vi "image_processing.vi"(5 "NG_rules":T3, 7 "parameter":T2={"image imshow"=FALSE, "side length (mm)"=0.0, "Main Range (Threshold)"={"Lower value"=73.0, "Upper value"=255.0}, "side velocity threshold"=0.0, "Sub Range (Threshold)"={"Lower value"=73.0, "Upper value"=255.0}, "close kernel size"=0.0, "open kernel size"=0.0, "side angle offest (threshold)"=0.0}, 11 "image":T1(plugin-control)) -> (0 "PASS":bool, 2 "NG code":dbl, 3 "display image":T1(plugin-control), 4 "angle offset":dbl)   [LabVIEW 2017]
uses:
  <vilib>/vision/NI_Vision_Development_Module.lvlib
panel:
  out "side angle offest":dbl
  out "side length (mm)":dbl
  out "ratio (cutting offest)":dbl
  out "damaged (mil)":dbl
  out "glitch (mil)":dbl
  out "open kernel size":dbl
  out "close kernel size":dbl
  in  "side velocity threshold":dbl
  out "Main Range (Threshold)":cluster{"Lower value":sgl, "Upper value":sgl}={"Lower value"=73.0, "Upper value"=255.0}
  out "image imshow":bool
  out "time image processing":u32
  out "time load image":u32
  out "Y Resolution":i32
  out "X Resolution":i32
  out "black image":T1(plugin-control)
  out "buffer image":T1(plugin-control)
  out "Sub Range (Threshold)":cluster{"Lower value":sgl, "Upper value":sgl}={"Lower value"=73.0, "Upper value"=255.0}
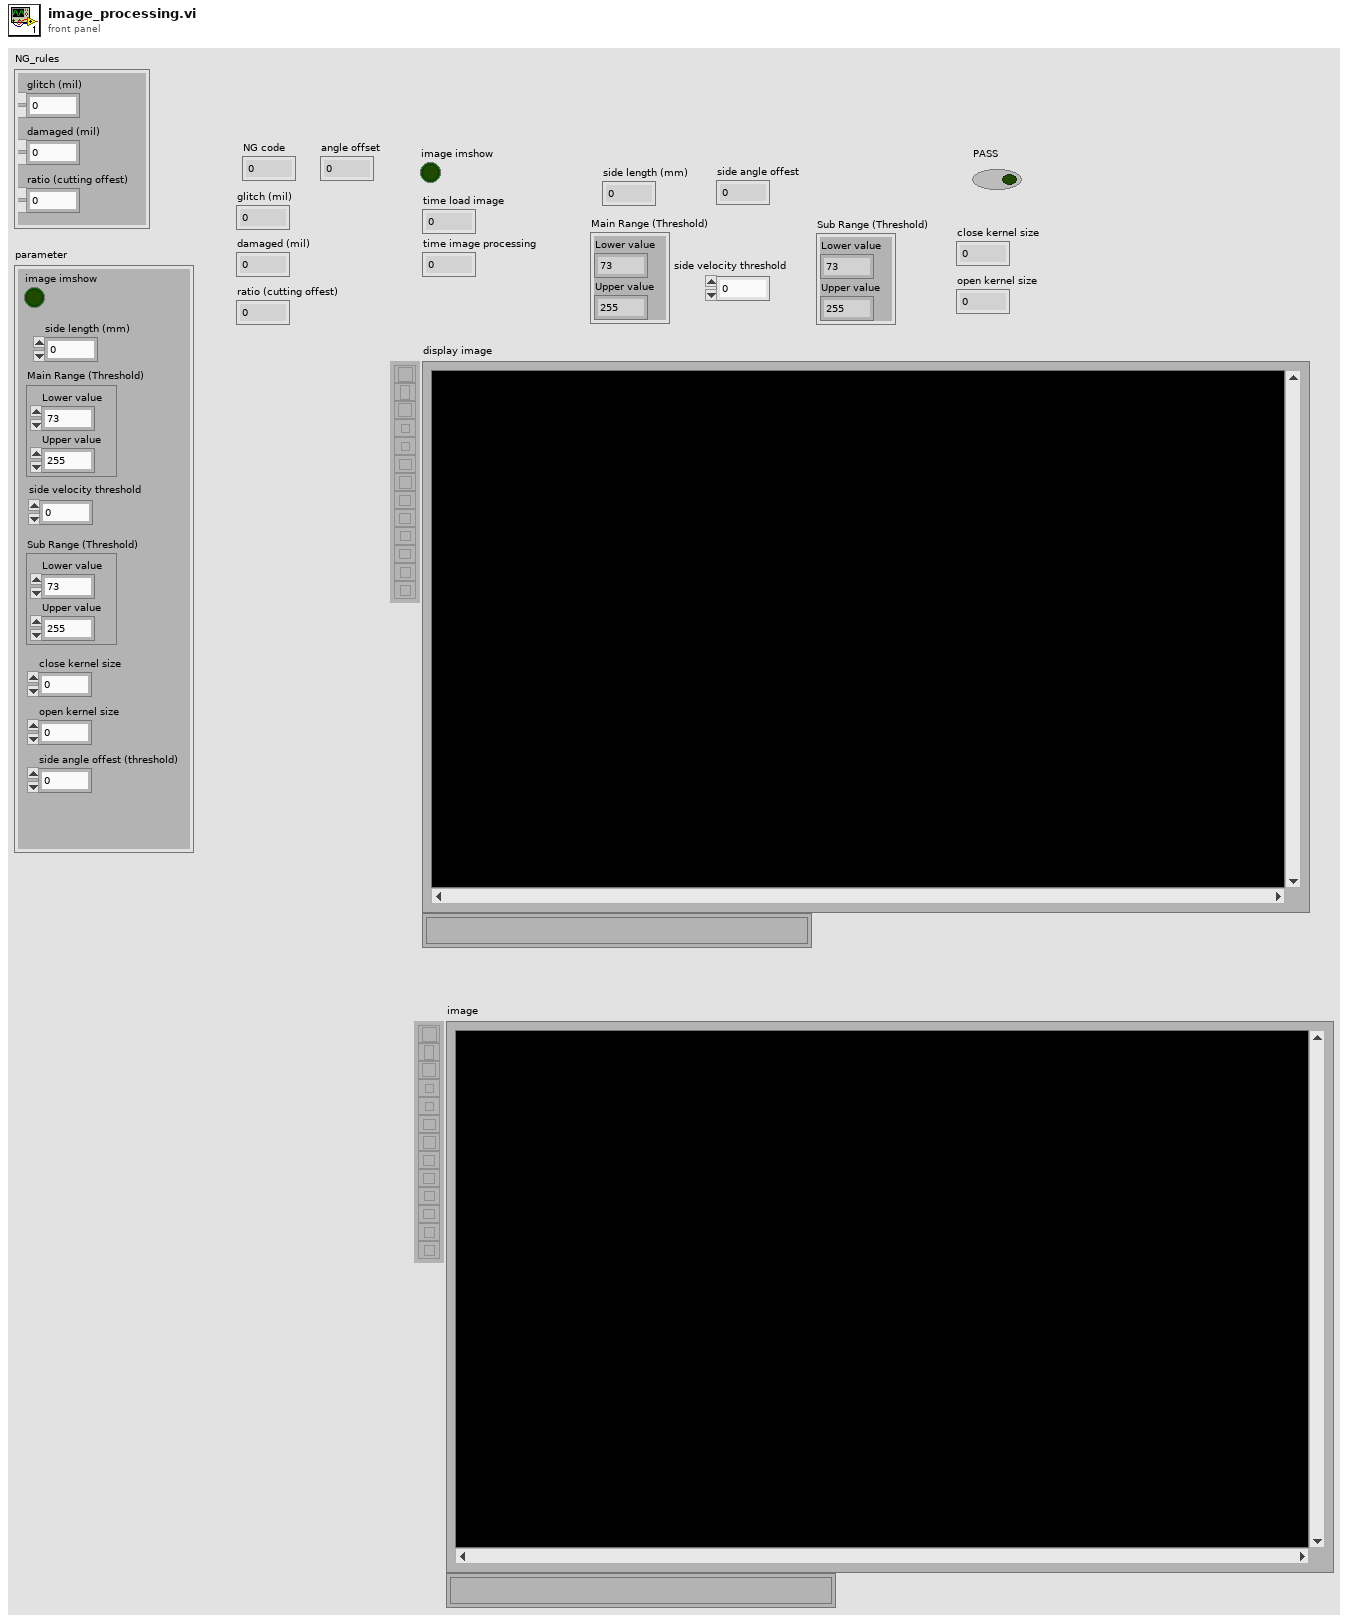
[diagram p1: front panel]
types:
  T1 = typedef "IMAQ Image.ctl" = refnum<image>
  T2 = cluster{"image imshow":bool, "side length (mm)":dbl, "Main Range (Threshold)":cluster{"Lower value":sgl, "Upper value":sgl}, "side velocity threshold":dbl, "Sub Range (Threshold)":cluster{"Lower value":sgl, "Upper value":sgl}, "close kernel size":dbl, "open kernel size":dbl, "side angle offest (threshold)":dbl}
  T3 = cluster{"glitch (mil)":dbl, "damaged (mil)":dbl, "ratio (cutting offest)":dbl}
  T4 = cluster{"Desired Font (Application)":enum16{"User-specified Font", "Application Font", "System Font", "Dialog Font"}, "[User-specified Font]":cluster{"Font Name":string, "Size":i16, "Strikeout?":bool, "Italic?":bool, "Underline?":bool, "Outline?":bool, "Shadow?":bool, "Bold?":bool, "Rotation Angle":dbl}, "Horizontal Alignment":i16, "Vertical Alignment":i16}
  T5 = enum32{"AutoM", "Close", "Dilate", "Erode", "Gradient", "Gradient out", "Gradient in", "Hit miss", "Open", "PClose", "POpen", "Thick", "Thin"}
  T6 = cluster{"Sigma":sgl, "HThresh":sgl, "LThres":sgl, "WindowSize":i32}
  T7 = cluster{"Number of Points":i32, "Open/Closed":i32, "Weight":dbl, "Contour Points":cluster{"X":dbl, "Y":dbl, "Curvature":dbl, "X Displacement":dbl, "Y Displacement":dbl}[]}[]
  T8 = cluster{"Left":i32, "Top":i32, "Right":i32, "Bottom":i32}
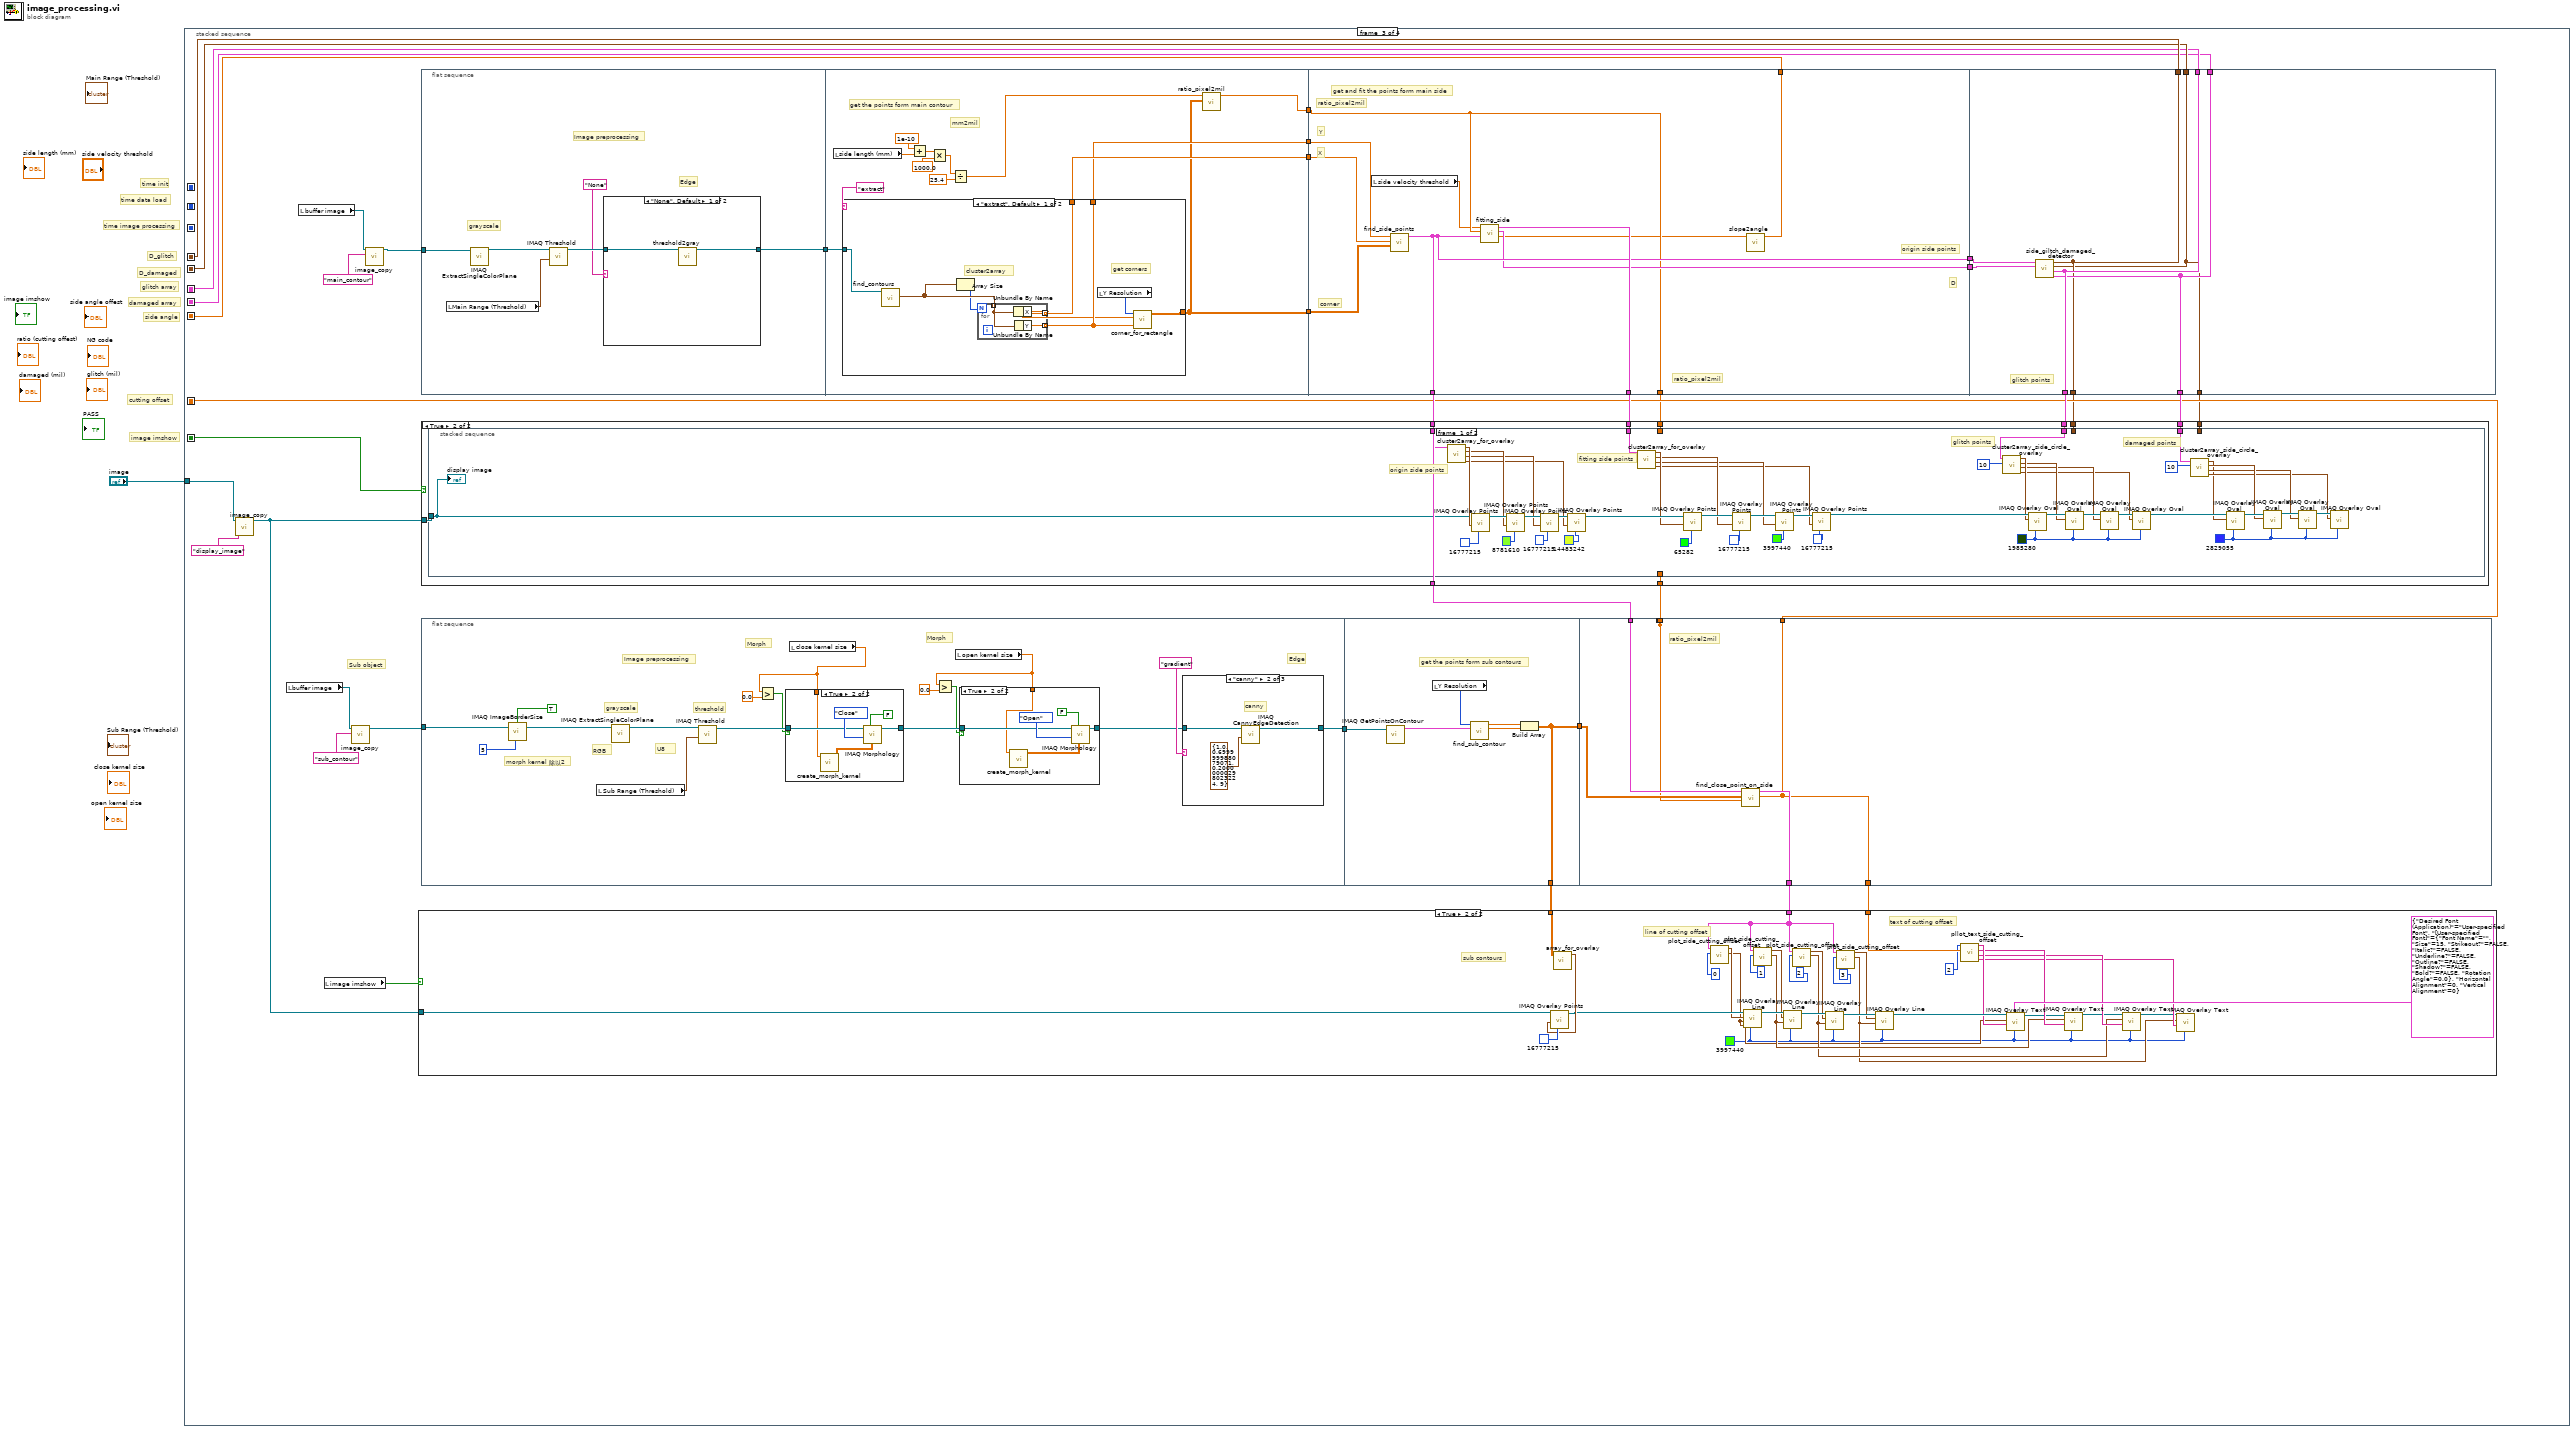
[diagram p0: block diagram]
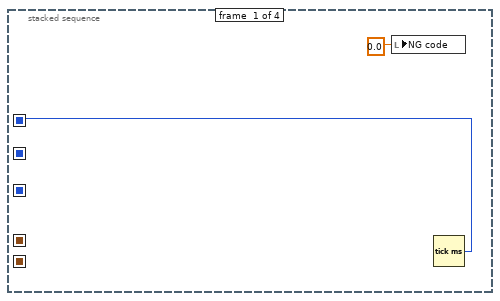
[diagram p2: hidden frame]
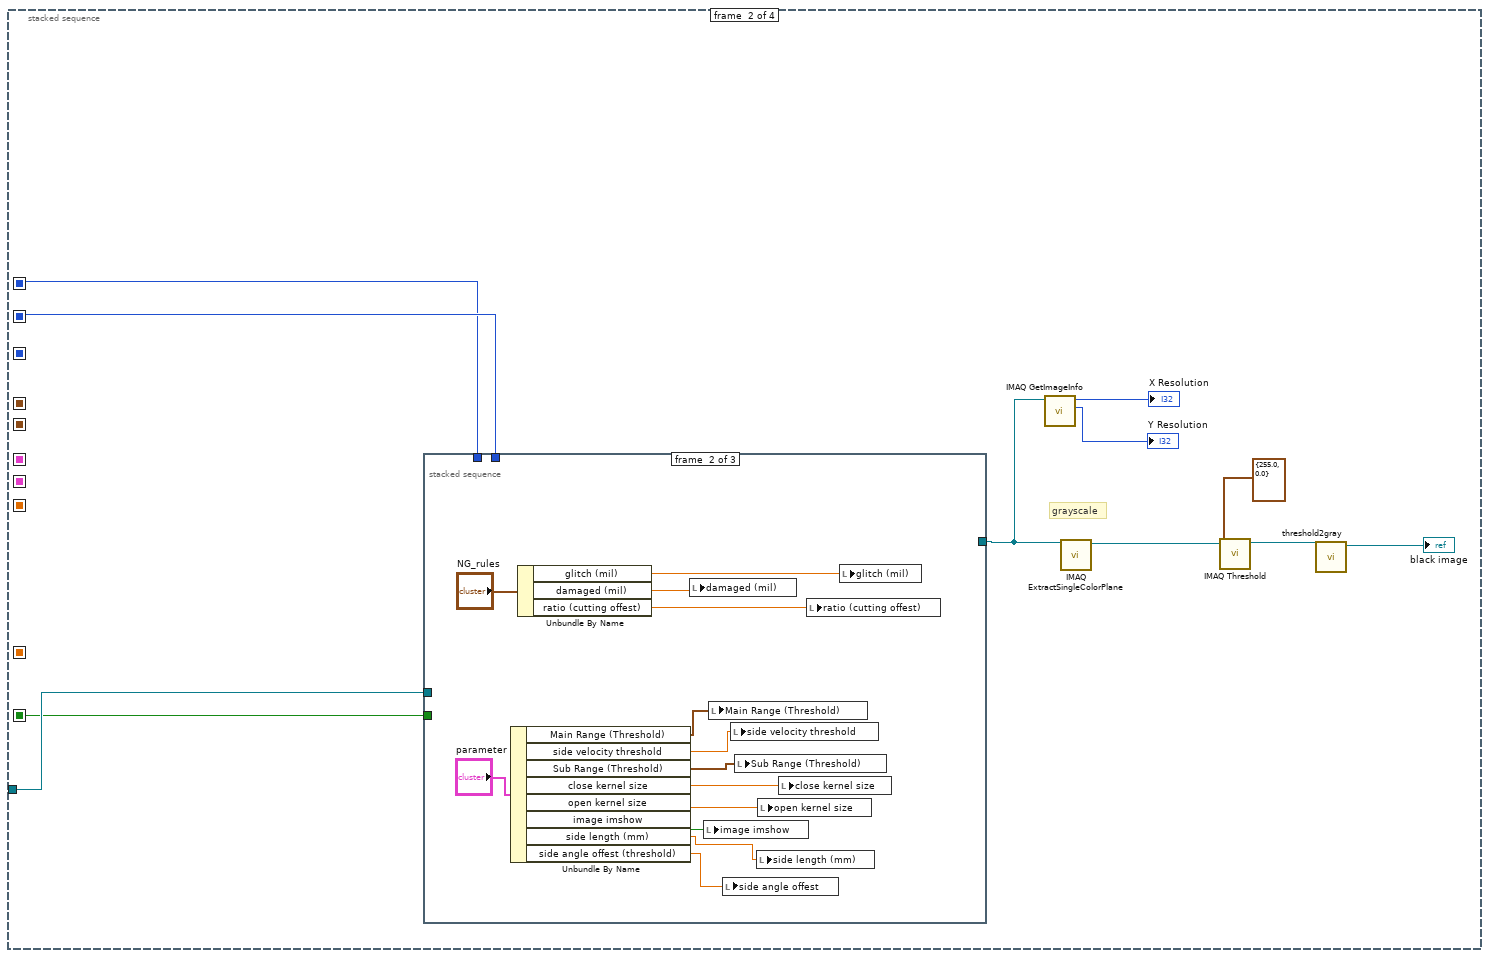
[diagram p3: hidden frame]
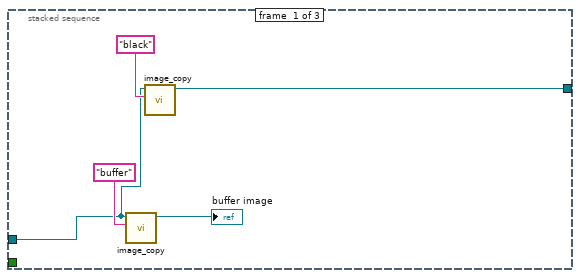
[diagram p4: hidden frame]
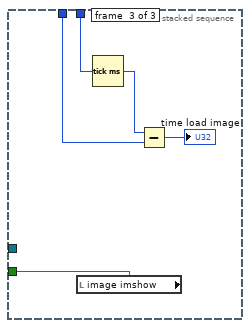
[diagram p5: hidden frame]
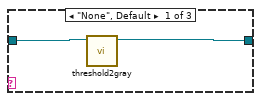
[diagram p9: hidden frame]
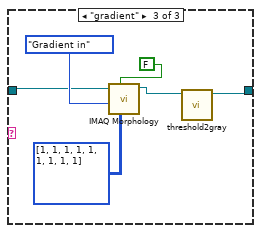
[diagram p10: hidden frame]
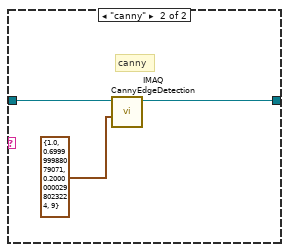
[diagram p11: hidden frame]
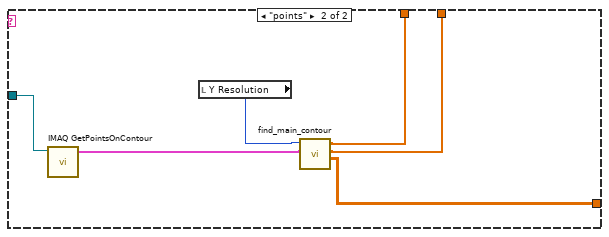
[diagram p12: hidden frame]
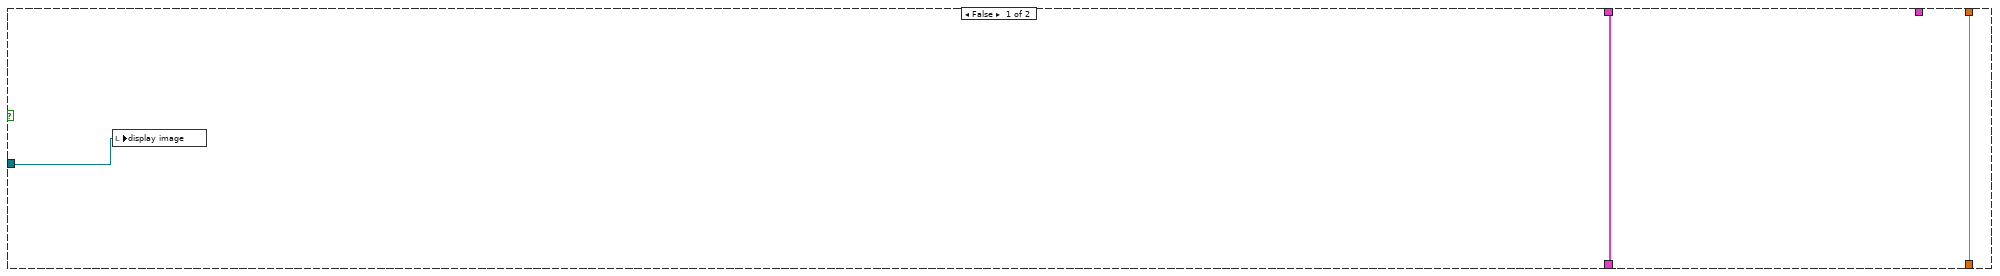
[diagram p13: hidden frame]
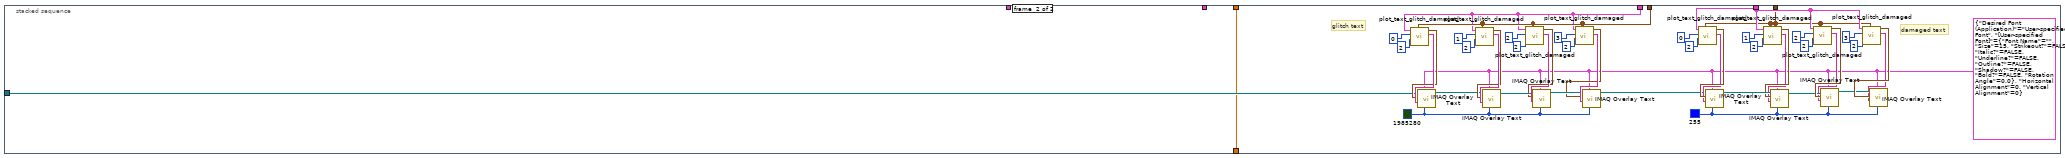
[diagram p14: hidden frame]
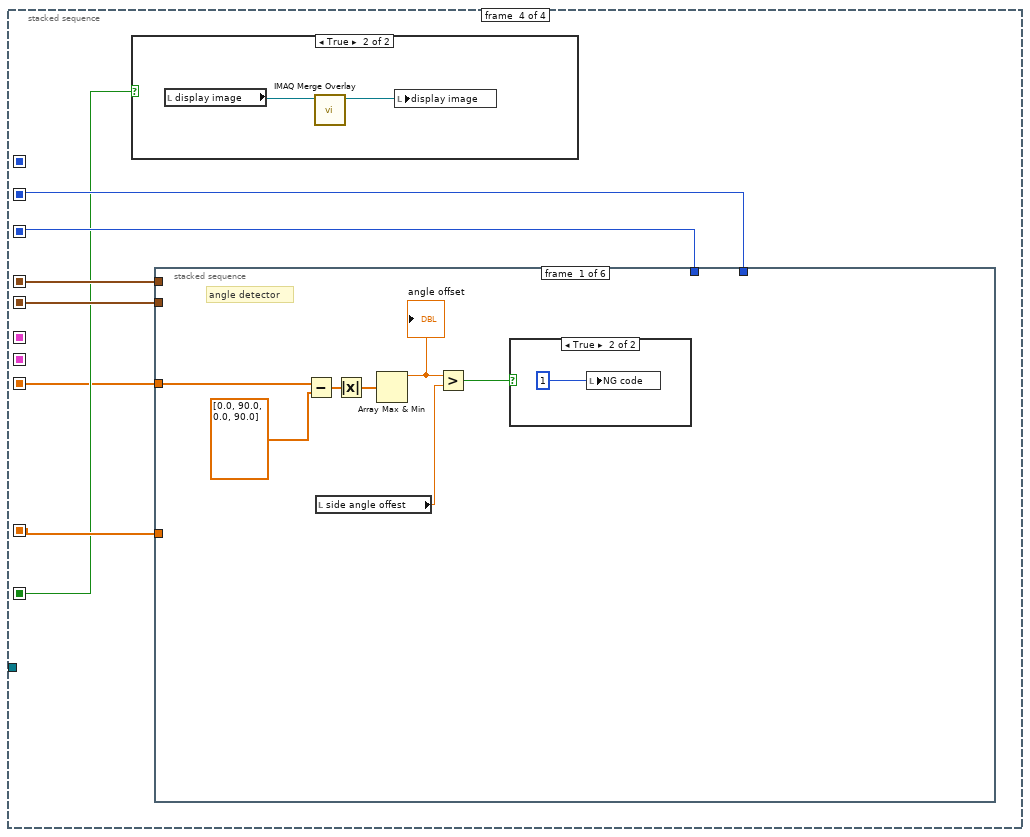
[diagram p15: hidden frame]
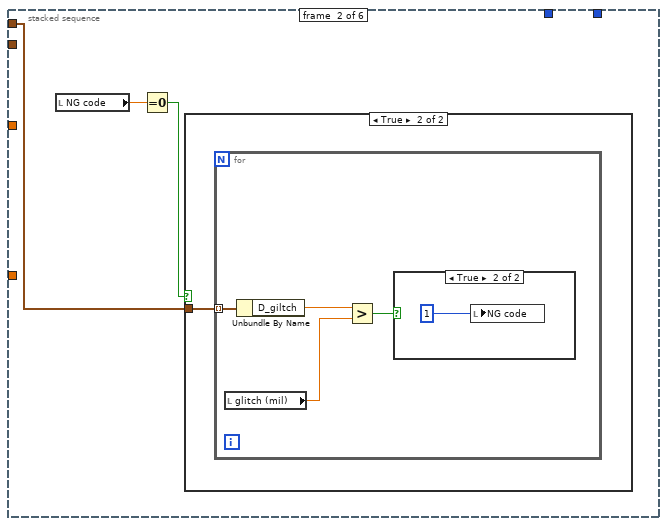
[diagram p18: hidden frame]
diagram:
  # "side angle"
  # "image imshow"
  # "cutting offset"
  # "damaged array"
  # "glitch array"
  # "D_damaged"
  # "D_glitch"
  # "time image processing"
  # "time data load"
  # "time init"
  n1 = stacked-sequence {
    seq-local: [w3 _ _ _] -> [_ w7 _ _]
    seq-local: [_ w8 _ _] -> [_ _ _ w330]
    seq-local: [_ _ _ w331] -> [_ _ _ _]
    seq-local: [_ _ w49 _] -> [_ _ _ w329]
    seq-local: [_ _ w48 _] -> [_ _ _ w328]
    seq-local: [_ _ w47 _] -> [_ _ _ _]
    seq-local: [_ _ w46 _] -> [_ _ _ _]
    seq-local: [_ _ w44 _] -> [_ _ _ w327]
    seq-local: [_ w4 _ _] -> [_ _ w38 w326]
    seq-local: [_ _ w37 _] -> [_ _ _ w325]
    tunnel: "image" -> [_ w9 w56 _]
    frame #0 {
      n2 = local write "NG code"(0.0 ("NG code")) -> ()
      n3 = Tick Count (ms)() -> (millisecond timer value=w3:u32)
    }
    frame #1 {
      # "grayscale"
      n4 = stacked-sequence {
        tunnel: [w17 _ _] -> w12
        tunnel: w9 -> [w16 _ _]
        tunnel: [_ _ w36] -> w8
        tunnel: w7 -> [_ _ w35]
        tunnel: [_ _ w33] -> w4
        frame #0 {
          n5 = call "image_copy.vi"("buffer name"="buffer" ("Image Name"), "image in"=w16) -> ("imgae out"=→"buffer image":T1)  [unwired: 9 in]
          n6 = call "image_copy.vi"("buffer name"="black" ("Image Name"), "image in"=w16) -> ("imgae out"=w17:T1)  [unwired: 9 in]
        }
        frame #1 {
          n7 = Unbundle By Name("parameter") -> ("Main Range (Threshold)"=w27:cluster{"Lower value":sgl, "Upper value":sgl}, "side velocity threshold"=w26:dbl, "Sub Range (Threshold)"=w25:cluster{"Lower value":sgl, "Upper value":sgl}, "close kernel size"=w24:dbl, "open kernel size"=w23:dbl, "image imshow"=w22:bool, "side length (mm)"=w21:dbl, "side angle offest (threshold)"=w20:dbl)
          n8 = Unbundle By Name("NG_rules") -> ("glitch (mil)"=w31:dbl, "damaged (mil)"=w30:dbl, "ratio (cutting offest)"=w29:dbl)
          n9 = local write "damaged (mil)"(w30) -> ()
          n10 = local write "image imshow"(w22) -> ()
          n11 = local write "Main Range (Threshold)"(w27) -> ()
          n12 = local write "side angle offest"(w20) -> ()
          n13 = local write "side velocity threshold"(w26) -> ()
          n14 = local write "Sub Range (Threshold)"(w25) -> ()
          n15 = local write "side length (mm)"(w21) -> ()
          n16 = local write "open kernel size"(w23) -> ()
          n17 = local write "close kernel size"(w24) -> ()
          n18 = local write "ratio (cutting offest)"(w29) -> ()
          n19 = local write "glitch (mil)"(w31) -> ()
        }
        frame #2 {
          n20 = local read "image imshow"() -> (w33:bool)
          n21 = Tick Count (ms)() -> (millisecond timer value=w36:u32)
          n22 = Subtract(x=w36, y=w35) -> (x-y=→"time load image":u32)
        }
      }
      n23 = call "IMAQ GetImageInfo"("Image"=w12) -> ("Y Resolution"=→"Y Resolution":i32, "X Resolution"=→"X Resolution":i32)  [unwired: 3 in, 6 out]
      n24 = call "IMAQ ExtractSingleColorPlane"("Image Src"=w12) -> ("Image Dst Out"=w14:T1)  [unwired: 3 in, 7 out]
      n25 = call "IMAQ Threshold"("Range"=cluster{"Lower value":sgl, "Upper value":sgl} {"Lower value"=255.0, "Upper value"=0.0}, "Image Src"=w14) -> ("Image Dst Out"=w6:T1)  [unwired: 4 in, 5 out]
      n26 = call "threshold2gray.vi"("threshold image"=w6) -> ("grayscale image"=→"black image":T1)  [unwired: 10 in]
    }
    frame #2 {
      # "Sub object"
      n27 = call "image_copy.vi"("buffer name"="display_image" ("Image Name"), "image in"=w56) -> ("imgae out"=w55:T1)  [unwired: 9 in]
      n28 = local read "buffer image"() -> (w65:T1)
      n29 = local read "buffer image"() -> (w73:T1)
      n30 = local read "image imshow"() -> (w52:bool)
      n31 = call "image_copy.vi"("buffer name"="sub_contour" ("Image Name"), "image in"=w65) -> ("imgae out"=w64:T1)  [unwired: 9 in]
      n32 = call "image_copy.vi"("buffer name"="main_contour" ("Image Name"), "image in"=w73) -> ("imgae out"=w72:T1)  [unwired: 9 in]
      n33 = case shown="True" w52 {
        tunnel: w55 -> [_ w75]
        tunnel: w54 -> [_ w105]
        tunnel: w53 -> [_ w97]
        tunnel: w43 -> [_ w90]
        frame False {
        }
        frame True {
          w76 = u32 3997440 ("Text Color (black)")
          # "text of cutting offset"
          # "line of cutting offset"
          # "sub contours"
          n34 = call "array_for_overlay.vi"("Array in"=w105) -> ("Array out"=w106:cluster{"X":i32, "Y":i32}[])  [unwired: 10 in]
          n35 = call "IMAQ Overlay Points"("Color"=u32 16777215, "Array of Points"=w106, "Image"=w75) -> ("Image Out"=w104:T1)  [unwired: 7 in, 1 out]
          n36 = call "plot_side_cutting_offset.vi"("index"=0, "coord cluster"=w97) -> ("End Point out"=w77:cluster{"X":i32, "Y":i32}, "Start Point out"=w87:cluster{"X":i32, "Y":i32})  [unwired: 8 in]
          n37 = call "IMAQ Overlay Line"("Color"=w76, "End Point"=w77, "Start Point"=w87, "Image"=w104) -> ("Image Out"=w103:T1)  [unwired: 6 in, 1 out]
          n38 = call "plot_side_cutting_offset.vi"("index"=1, "coord cluster"=w97) -> ("End Point out"=w80:cluster{"X":i32, "Y":i32}, "Start Point out"=w92:cluster{"X":i32, "Y":i32})  [unwired: 8 in]
          n39 = call "IMAQ Overlay Line"("Color"=w76, "End Point"=w80, "Start Point"=w92, "Image"=w103) -> ("Image Out"=w102:T1)  [unwired: 6 in, 1 out]
          n40 = call "plot_side_cutting_offset.vi"("index"=2, "coord cluster"=w97) -> ("End Point out"=w79:cluster{"X":i32, "Y":i32}, "Start Point out"=w93:cluster{"X":i32, "Y":i32})  [unwired: 8 in]
          n41 = call "IMAQ Overlay Line"("Color"=w76, "End Point"=w79, "Start Point"=w93, "Image"=w102) -> ("Image Out"=w101:T1)  [unwired: 6 in, 1 out]
          n42 = call "plot_side_cutting_offset.vi"("index"=3, "coord cluster"=w97) -> ("End Point out"=w78:cluster{"X":i32, "Y":i32}, "Start Point out"=w94:cluster{"X":i32, "Y":i32})  [unwired: 8 in]
          n43 = call "IMAQ Overlay Line"("Color"=w76, "End Point"=w78, "Start Point"=w94, "Image"=w101) -> ("Image Out"=w95:T1)  [unwired: 6 in, 1 out]
          n44 = call "pllot_text_side_cutting_offset.vi"("D cutting offset array"=w90, "precision"=2 ("index")) -> ("Left side length"=w84:string, "Bottom side length"=w85:string, "Right side length"=w86:string, "Top side length"=w88:string)  [unwired: 6 in]
          n45 = call "IMAQ Overlay Text"("Text Color (black)"=w76, "Font, Size & Style"=T4 {"Desired Font (Application)"=enum."User-specified Font", "[User-specified Font]"={"Font Name"="", "Size"=15, "Strikeout?"=FALSE, "Italic?"=FALSE, "Underline?"=FALSE, "Outline?"=FALSE, "Shadow?"=FALSE, "Bold?"=FALSE, "Rotation Angle"=0.0}, "Horizontal Alignment"=0, "Vertical Alignment"=0}, "String"=w88, "Origin"=w77, "Image"=w95) -> ("Image Out"=w83:T1)  [unwired: 5 in, 1 out]
          n46 = call "IMAQ Overlay Text"("Text Color (black)"=w76, "String"=w86, "Origin"=w80, "Image"=w83) -> ("Image Out"=w82:T1)  [unwired: 6 in, 1 out]
          n47 = call "IMAQ Overlay Text"("Text Color (black)"=w76, "String"=w85, "Origin"=w79, "Image"=w82) -> ("Image Out"=w81:T1)  [unwired: 6 in, 1 out]
          n48 = call "IMAQ Overlay Text"("Text Color (black)"=w76, "String"=w84, "Origin"=w78, "Image"=w81) -> ()  [unwired: 6 in, 2 out]
        }
      }
      n49 = flat-sequence {
        tunnel: w72 -> [w166]
        tunnel: [w163] -> w71
        tunnel: w71 -> [w183]
        tunnel: [w177] -> w70
        tunnel: [w182] -> w68
        tunnel: [w181] -> w67
        tunnel: [w175] -> w59
        tunnel: w70 -> [w210]
        tunnel: [w206] -> w69
        tunnel: w68 -> [w209]
        tunnel: w67 -> [w208]
        tunnel: [w207] -> w62
        tunnel: w59 -> [w204]
        tunnel: [w206] -> w51
        tunnel: [w205] -> w50
        tunnel: [w204] -> w40
        tunnel: [w201] -> w37
        tunnel: [w214] -> w61
        tunnel: [w213] -> w60
        tunnel: w51 -> [w216]
        tunnel: w50 -> [w215]
        tunnel: [w214] -> w47
        tunnel: [w213] -> w46
        tunnel: [w212] -> w49
        tunnel: [w211] -> w48
        tunnel: [w212] -> w42
        tunnel: [w211] -> w41
        frame #0 {
          # "Image preprocessing"
          # "grayscale"
          # "Edge"
          n50 = local read "Main Range (Threshold)"() -> (w161:cluster{"Lower value":sgl, "Upper value":sgl})
          n51 = call "IMAQ ExtractSingleColorPlane"("Image Src"=w166) -> ("Image Dst Out"=w165:T1)  [unwired: 3 in, 7 out]
          n52 = call "IMAQ Threshold"("Range"=w161, "Image Src"=w165) -> ("Image Dst Out"=w164:T1)  [unwired: 4 in, 5 out]
          n53 = case shown="\"None\", Default" "None" {
            tunnel: [w167 w171] -> w163
            tunnel: w164 -> [w168 w170]
            frame "None", Default {
              n54 = call "threshold2gray.vi"("threshold image"=w168) -> ("grayscale image"=w167:T1)  [unwired: 10 in]
            }
            frame "canny" {
              # "canny"
              n55 = call "IMAQ CannyEdgeDetection"("Image Src"=w170, "Filter Parameters"=T6 {"Sigma"=1.0, "HThresh"=0.7, "LThres"=0.2, "WindowSize"=9}) -> ("Image Dst Out"=w171:T1)  [unwired: 2 in, 5 out]
            }
          }
        }
        frame #1 {
          # "mm2mil"
          # "get the points form main contour"
          n56 = local read "side length (mm)"() -> (w172:dbl)
          n57 = case shown="\"extract\", Default" "extract" {
            tunnel: w183 -> [w187 w200]
            tunnel: [w188 w195] -> w177
            tunnel: [w186 w196] -> w181
            tunnel: [w185 w197] -> w182
            frame "extract", Default {
              # "get corners"
              # "cluster2array"
              n58 = call "find_contours.vi"("image in"=w187) -> ("Source Image Points"=w191:cluster{"X":dbl, "Y":dbl}[])  [unwired: 9 in, 1 out]
              n59 = Array Size(array=w191) -> (size(s)=w189:i32)
              n60 = for {
                N: w189 -> [_]
                tunnel: w191 -> [w193] mode=indexing
                tunnel: [w194] -> w185 mode=indexing
                tunnel: [w192] -> w186 mode=indexing
                n61 = Unbundle By Name(w193) -> ("X"=w194:dbl)
                n62 = Unbundle By Name(w193) -> ("Y"=w192:dbl)
              }
              n63 = local read "Y Resolution"() -> (w190:i32)
              n64 = call "corner_for_rectangle.vi"("Y"=w186, "X"=w185, "Y Resolution"=w190) -> ("corner"=w188:dbl[][])  [unwired: 7 in, 1 out]
            }
            frame "points" {
              n65 = call "IMAQ GetPointsOnContour"("Image (Edge Image)"=w200) -> ("Segment Information"=w198:T7)  [unwired: 3 in, 2 out]
              n66 = local read "Y Resolution"() -> (w199:i32)
              n67 = call "find_main_contour.vi"("Segment Information"=w198, "Y Resolution"=w199) -> ("max corner"=w195:dbl[][], "Y"=w196:dbl[], "X"=w197:dbl[])  [unwired: 7 in]
            }
          }
          n68 = Add(x=1e-10, y=w172) -> (x+y=w173:dbl)
          n69 = Multiply(x=w173, y=1000.0) -> (x*y=w179:dbl)
          n70 = Divide(x=w179, y=25.4) -> (x/y=w176:dbl)
          n71 = call "ratio_pixel2mil.vi"("max corner in"=w177, "side length (mm)"=w176) -> ("ratio"=w175:dbl)  [unwired: 9 in]
        }
        frame #2 {
          # "ratio_pixel2mil"
          # "origin side points"
          # "D"
          # "corner"
          # "X"
          # "Y"
          # "ratio_pixel2mil"
          # "get and fit the points form main side"
          n72 = local read "side velocity threshold"() -> (w203:dbl)
          n73 = call "find_side_points.vi"("corner"=w210, "X  coords array"=w209, "Y coords array"=w208) -> ("side of clusters"=w206:cluster{"Array out":dbl[][]}[])  [unwired: 8 in]
          n74 = call "fitting_side.vi"("side of clusters"=w206, "ratio"=w204, "side velocity threshold"=w203) -> ("slope array"=w202:dbl[], "D of clusters"=w205:cluster{"D":ext[]}[], "fitting clusters"=w207:cluster{"fitting array":dbl[][]}[])  [unwired: 6 in]
          n75 = call "slope2angle.vi"("slope array"=w202) -> ("x/y"=w201:dbl[])  [unwired: 10 in]
        }
        frame #3 {
          # "glitch points"
          n76 = call "side_giltch_damaged_detector.vi"("D of clusters"=w215, "side of clusters"=w216) -> ("damaged clusters"=w213:cluster{"damaged coord":dbl[]}[], "giltch of clusters"=w214:cluster{"giltch_coord":dbl[]}[], "D damaged of clusters"=w211:cluster{"D_damaged":ext}[], "D giltch of clusters"=w212:cluster{"D_giltch":ext}[])  [unwired: 6 in]
        }
      }
      n77 = flat-sequence {
        tunnel: w64 -> [w121]
        tunnel: [w117] -> w63
        tunnel: w63 -> [w155]
        tunnel: [w150] -> w58
        tunnel: [w150] -> w54
        tunnel: w58 -> [w160]
        tunnel: [w159] -> w53
        tunnel: w45 -> [w158]
        tunnel: [w156] -> w44
        tunnel: [w156] -> w43
        tunnel: [w157] -> _
        tunnel: w39 -> [w157]
        frame #0 {
          # "Morph"
          # "Image preprocessing"
          # "Morph"
          # "morph kernel 除以2"
          # "Edge"
          # "U8"
          # "RGB"
          # "threshold"
          # "grayscale"
          n78 = call "IMAQ ImageBorderSize"("Get/Set Status? (Set)"=TRUE, "Image"=w121, "Image border size in"=5) -> ("Image Out"=w120:T1)  [unwired: 1 in, 2 out]
          n79 = local read "Sub Range (Threshold)"() -> (w110:cluster{"Lower value":sgl, "Upper value":sgl})
          n80 = call "IMAQ ExtractSingleColorPlane"("Image Src"=w120) -> ("Image Dst Out"=w124:T1)  [unwired: 3 in, 7 out]
          n81 = call "IMAQ Threshold"("Range"=w110, "Image Src"=w124) -> ("Image Dst Out"=w122:T1)  [unwired: 4 in, 5 out]
          n82 = local read "close kernel size"() -> (w109:dbl)
          n83 = Greater?(x=w109, y=0.0) -> (0:w114:bool)
          n84 = case shown="True" w114 {
            tunnel: w122 -> [w132 w137]
            tunnel: [w132 w136] -> w115
            tunnel: w109 -> [_ w135]
            frame False {
            }
            frame True {
              n85 = call "create_morph_kernel.vi"("kernel size"=w135) -> ("kernel"=w134:dbl[][])  [unwired: 10 in]
              n86 = call "IMAQ Morphology"("Structuring Element"=w134, "Square/Hexa (Square)"=FALSE, "Operation"=T5."Close", "Image Src"=w137) -> ("Image Dst Out"=w136:T1)  [unwired: 3 in, 4 out]
            }
          }
          n87 = local read "open kernel size"() -> (w108:dbl)
          n88 = Greater?(x=w108, y=0.0) -> (0:w111:bool)
          n89 = case shown="True" w111 {
            tunnel: [w125 w130] -> w116
            tunnel: w115 -> [w125 w129]
            tunnel: w108 -> [_ w126]
            frame False {
            }
            frame True {
              n90 = call "create_morph_kernel.vi"("kernel size"=w126) -> ("kernel"=w127:dbl[][])  [unwired: 10 in]
              n91 = call "IMAQ Morphology"("Structuring Element"=w127, "Square/Hexa (Square)"=FALSE, "Operation"=T5."Open", "Image Src"=w129) -> ("Image Dst Out"=w130:T1)  [unwired: 3 in, 4 out]
            }
          }
          n92 = case shown="\"canny\"" "gradient" {
            tunnel: [w139 w143 w144] -> w117
            tunnel: w116 -> [w140 w142 w146]
            frame "None", Default {
              n93 = call "threshold2gray.vi"("threshold image"=w140) -> ("grayscale image"=w139:T1)  [unwired: 10 in]
            }
            frame "canny" {
              # "canny"
              n94 = call "IMAQ CannyEdgeDetection"("Image Src"=w142, "Filter Parameters"=T6 {"Sigma"=1.0, "HThresh"=0.7, "LThres"=0.2, "WindowSize"=9}) -> ("Image Dst Out"=w143:T1)  [unwired: 2 in, 5 out]
            }
            frame "gradient" {
              n95 = call "IMAQ Morphology"("Structuring Element"=i32[][] [[1, 1, 1], [1, 1, 1], [1, 1, 1]], "Square/Hexa (Square)"=FALSE, "Operation"=T5."Gradient in", "Image Src"=w146) -> ("Image Dst Out"=w145:T1)  [unwired: 3 in, 4 out]
              n96 = call "threshold2gray.vi"("threshold image"=w145) -> ("grayscale image"=w144:T1)  [unwired: 10 in]
            }
          }
        }
        frame #1 {
          # "get the points form sub contours"
          n97 = call "IMAQ GetPointsOnContour"("Image (Edge Image)"=w155) -> ("Segment Information"=w154:T7)  [unwired: 3 in, 2 out]
          n98 = local read "Y Resolution"() -> (w153:i32)
          n99 = call "find_sub_contour.vi"("Segment Information"=w154, "Y Resolution"=w153) -> ("Y"=w151:dbl[], "X"=w152:dbl[])  [unwired: 8 in]
          n100 = Build Array(w152, w151) -> (w150:dbl[][])
        }
        frame #2 {
          # "ratio_pixel2mil"
          n101 = call "find_close_point_on_side.vi"("ratio_pixel2mil"=w157, "Array"=w160, "fitting clusters"=w158) -> ("D cutting offset array"=w156:ext[], "coord cluster"=w159:cluster{dbl[][]}[])  [unwired: 7 in]
        }
      }
      n102 = case shown="True" w38 {
        tunnel: w55 -> [w218 w228]
        tunnel: w69 -> [w217 w220]
        tunnel: w62 -> [_ w225]
        tunnel: w61 -> [_ w226]
        tunnel: w60 -> [_ w227]
        tunnel: [w217 w220] -> w45
        tunnel: w42 -> [_ w224]
        tunnel: w41 -> [_ w223]
        tunnel: w40 -> [w219 w222]
        tunnel: [w219 w221] -> w39
        frame False {
          n103 = local write "display image"(w218) -> ()
        }
        frame True {
          n104 = stacked-sequence {
            tunnel: w228 -> [w229 w320]
            tunnel: w220 -> [w251 _]
            tunnel: w227 -> [w236 w283]
            tunnel: w226 -> [w231 w305]
            tunnel: w225 -> [w230 _]
            tunnel: w224 -> [_ w307]
            tunnel: w223 -> [_ w282]
            tunnel: w222 -> [_ w278]
            tunnel: [_ w278] -> w221
            frame #0 {
              w253 = u32 2829055 ("Color")
              w254 = u32 1985280 ("Color")
              # "damaged points"
              # "glitch points"
              # "fitting side points"
              # "origin side points"
              n105 = call "cluster2array_for_overlay.vi"("side of clusters"=w251) -> ("Left side points"=w247:cluster{"X":i32, "Y":i32}[], "Bottom side points"=w248:cluster{"X":i32, "Y":i32}[], "Right side points"=w249:cluster{"X":i32, "Y":i32}[], "Top side points"=w250:cluster{"X":i32, "Y":i32}[])  [unwired: 7 in]
              n106 = call "IMAQ Overlay Points"("Color"=u32 16777215, "Array of Points"=w250, "Image"=w229) -> ("Image Out"=w273:T1)  [unwired: 7 in, 1 out]
              n107 = call "IMAQ Overlay Points"("Color"=u32 8781610, "Array of Points"=w249, "Image"=w273) -> ("Image Out"=w275:T1)  [unwired: 7 in, 1 out]
              n108 = call "IMAQ Overlay Points"("Color"=u32 16777215, "Array of Points"=w248, "Image"=w275) -> ("Image Out"=w274:T1)  [unwired: 7 in, 1 out]
              n109 = call "IMAQ Overlay Points"("Color"=u32 14483242, "Array of Points"=w247, "Image"=w274) -> ("Image Out"=w262:T1)  [unwired: 7 in, 1 out]
              n110 = call "cluster2array_for_overlay.vi"("side of clusters"=w230) -> ("Left side points"=w243:cluster{"X":i32, "Y":i32}[], "Bottom side points"=w244:cluster{"X":i32, "Y":i32}[], "Right side points"=w245:cluster{"X":i32, "Y":i32}[], "Top side points"=w246:cluster{"X":i32, "Y":i32}[])  [unwired: 7 in]
              n111 = call "IMAQ Overlay Points"("Color"=u32 65282, "Array of Points"=w246, "Image"=w262) -> ("Image Out"=w266:T1)  [unwired: 7 in, 1 out]
              n112 = call "IMAQ Overlay Points"("Color"=u32 16777215, "Array of Points"=w245, "Image"=w266) -> ("Image Out"=w264:T1)  [unwired: 7 in, 1 out]
              n113 = call "IMAQ Overlay Points"("Color"=u32 3997440, "Array of Points"=w244, "Image"=w264) -> ("Image Out"=w265:T1)  [unwired: 7 in, 1 out]
              n114 = call "IMAQ Overlay Points"("Color"=u32 16777215, "Array of Points"=w243, "Image"=w265) -> ("Image Out"=w252:T1)  [unwired: 7 in, 1 out]
              n115 = call "cluster2array_side_circle_overlay.vi"("radius"=10 ("index"), "giltch of clusters"=w231) -> ("Left side points"=w239:T8, "Bottom side points"=w240:T8, "Right side points"=w241:T8, "Top side points"=w242:T8)  [unwired: 6 in]
              n116 = call "IMAQ Overlay Oval"("Color"=w254, "Bounding Rectangle"=w242, "Image"=w252) -> ("Image Out"=w261:T1)  [unwired: 7 in, 1 out]
              n117 = call "IMAQ Overlay Oval"("Color"=w254, "Bounding Rectangle"=w241, "Image"=w261) -> ("Image Out"=w260:T1)  [unwired: 7 in, 1 out]
              n118 = call "IMAQ Overlay Oval"("Color"=w254, "Bounding Rectangle"=w240, "Image"=w260) -> ("Image Out"=w259:T1)  [unwired: 7 in, 1 out]
              n119 = call "IMAQ Overlay Oval"("Color"=w254, "Bounding Rectangle"=w239, "Image"=w259) -> ("Image Out"=w255:T1)  [unwired: 7 in, 1 out]
              n120 = call "cluster2array_side_circle_overlay.vi"("radius"=10 ("index"), "giltch of clusters"=w236) -> ("Left side points"=w233:T8, "Bottom side points"=w234:T8, "Right side points"=w235:T8, "Top side points"=w232:T8)  [unwired: 6 in]
              n121 = call "IMAQ Overlay Oval"("Color"=w253, "Bounding Rectangle"=w232, "Image"=w255) -> ("Image Out"=w256:T1)  [unwired: 7 in, 1 out]
              n122 = call "IMAQ Overlay Oval"("Color"=w253, "Bounding Rectangle"=w235, "Image"=w256) -> ("Image Out"=w257:T1)  [unwired: 7 in, 1 out]
              n123 = call "IMAQ Overlay Oval"("Color"=w253, "Bounding Rectangle"=w234, "Image"=w257) -> ("Image Out"=w258:T1)  [unwired: 7 in, 1 out]
              n124 = call "IMAQ Overlay Oval"("Color"=w253, "Bounding Rectangle"=w233, "Image"=w258) -> ()  [unwired: 7 in, 2 out]
              "display image" <- w229
            }
            frame #1 {
              w277 = u32 1985280 ("Color")
              w280 = u32 255 ("Text Color (black)")
              w281 = T4 {"Desired Font (Application)"=enum."User-specified Font", "[User-specified Font]"={"Font Name"="", "Size"=15, "Strikeout?"=FALSE, "Italic?"=FALSE, "Underline?"=FALSE, "Outline?"=FALSE, "Shadow?"=FALSE, "Bold?"=FALSE, "Rotation Angle"=0.0}, "Horizontal Alignment"=0, "Vertical Alignment"=0} ("Font, Size & Style")
              # "damaged text"
              # "glitch text"
              n125 = call "plot_text_glitch_damaged.vi"("D of clusters"=w307, "precision"=2 ("index (page)"), "index"=0 ("index (page)"), "array clusters"=w305) -> ("string"=w322:string, "Origin"=w321:cluster{"X":i32, "Y":i32})  [unwired: 6 in]
              n126 = call "IMAQ Overlay Text"("Text Color (black)"=w277, "Font, Size & Style"=w281, "String"=w322, "Origin"=w321, "Image"=w320) -> ("Image Out"=w315:T1)  [unwired: 5 in, 1 out]
              n127 = call "plot_text_glitch_damaged.vi"("D of clusters"=w307, "precision"=2 ("index (page)"), "index"=1 ("index (page)"), "array clusters"=w305) -> ("string"=w319:string, "Origin"=w316:cluster{"X":i32, "Y":i32})  [unwired: 6 in]
              n128 = call "IMAQ Overlay Text"("Text Color (black)"=w277, "Font, Size & Style"=w281, "String"=w319, "Origin"=w316, "Image"=w315) -> ("Image Out"=w308:T1)  [unwired: 5 in, 1 out]
              n129 = call "plot_text_glitch_damaged.vi"("D of clusters"=w307, "precision"=2 ("index (page)"), "index"=2 ("index (page)"), "array clusters"=w305) -> ("string"=w312:string, "Origin"=w303:cluster{"X":i32, "Y":i32})  [unwired: 6 in]
              n130 = call "IMAQ Overlay Text"("Text Color (black)"=w277, "Font, Size & Style"=w281, "String"=w312, "Origin"=w303, "Image"=w308) -> ("Image Out"=w306:T1)  [unwired: 5 in, 1 out]
              n131 = call "plot_text_glitch_damaged.vi"("D of clusters"=w307, "precision"=2 ("index (page)"), "index"=3 ("index (page)"), "array clusters"=w305) -> ("string"=w311:string, "Origin"=w304:cluster{"X":i32, "Y":i32})  [unwired: 6 in]
              n132 = call "IMAQ Overlay Text"("Text Color (black)"=w277, "Font, Size & Style"=w281, "String"=w311, "Origin"=w304, "Image"=w306) -> ("Image Out"=w279:T1)  [unwired: 5 in, 1 out]
              n133 = call "plot_text_glitch_damaged.vi"("D of clusters"=w282, "precision"=2 ("index (page)"), "index"=0 ("index (page)"), "array clusters"=w283) -> ("string"=w286:string, "Origin"=w287:cluster{"X":i32, "Y":i32})  [unwired: 6 in]
              n134 = call "IMAQ Overlay Text"("Text Color (black)"=w280, "Font, Size & Style"=w281, "String"=w286, "Origin"=w287, "Image"=w279) -> ("Image Out"=w292:T1)  [unwired: 5 in, 1 out]
              n135 = call "plot_text_glitch_damaged.vi"("D of clusters"=w282, "precision"=2 ("index (page)"), "index"=1 ("index (page)"), "array clusters"=w283) -> ("string"=w288:string, "Origin"=w291:cluster{"X":i32, "Y":i32})  [unwired: 6 in]
              n136 = call "IMAQ Overlay Text"("Text Color (black)"=w280, "Font, Size & Style"=w281, "String"=w288, "Origin"=w291, "Image"=w292) -> ("Image Out"=w299:T1)  [unwired: 5 in, 1 out]
              n137 = call "plot_text_glitch_damaged.vi"("D of clusters"=w282, "precision"=2 ("index (page)"), "index"=2 ("index (page)"), "array clusters"=w283) -> ("string"=w295:string, "Origin"=w302:cluster{"X":i32, "Y":i32})  [unwired: 6 in]
              n138 = call "IMAQ Overlay Text"("Text Color (black)"=w280, "Font, Size & Style"=w281, "String"=w295, "Origin"=w302, "Image"=w299) -> ("Image Out"=w300:T1)  [unwired: 5 in, 1 out]
              n139 = call "plot_text_glitch_damaged.vi"("D of clusters"=w282, "precision"=2 ("index (page)"), "index"=3 ("index (page)"), "array clusters"=w283) -> ("string"=w296:string, "Origin"=w301:cluster{"X":i32, "Y":i32})  [unwired: 6 in]
              n140 = call "IMAQ Overlay Text"("Text Color (black)"=w280, "Font, Size & Style"=w281, "String"=w296, "Origin"=w301, "Image"=w300) -> ()  [unwired: 5 in, 2 out]
            }
          }
        }
      }
    }
    frame #3 {
      n141 = case shown="True" w326 {
        frame False {
        }
        frame True {
          n142 = local read "display image"() -> (w333:T1)
          n143 = call "IMAQ Merge Overlay"("Image Src"=w333) -> ("Image Dst Out"=w332:T1)  [unwired: 9 in, 1 out]
          n144 = local write "display image"(w332) -> ()
        }
      }
      n145 = stacked-sequence {
        tunnel: [_ _ _ _ _ w397] -> w331
        tunnel: w330 -> [_ _ _ _ _ w396]
        tunnel: w329 -> [_ w344 _ _ _ _]
        tunnel: w328 -> [_ _ w351 _ _ _]
        tunnel: w327 -> [_ _ _ w360 _ _]
        tunnel: w325 -> [w340 _ _ _ _ _]
        frame #0 {
          # "angle detector"
          n146 = Subtract(x=w340, y=dbl[] [0.0, 90.0, 0.0, 90.0] ("x/y")) -> (x-y=w338:dbl[])
          n147 = local read "side angle offest"() -> (w336:dbl)
          n148 = Absolute Value(x=w338) -> (abs(x)=w337:dbl[])
          n149 = Array Max & Min(array=w337) -> (max value=w335:dbl)  [unwired: 3 out]
          "angle offset" <- w335
          n150 = Greater?(x=w335, y=w336) -> (0:w334:bool)
          n151 = case shown="True" w334 {
            frame False {
            }
            frame True {
              n152 = local write "NG code"(1) -> ()
            }
          }
        }
        frame #1 {
          n153 = local read "NG code"() -> (w343:dbl)
          n154 = Equal To 0?(x=w343) -> (x = 0?=w342:bool)
          n155 = case shown="True" w342 {
            tunnel: w344 -> [_ w345]
            frame False {
            }
            frame True {
              n156 = for {
                tunnel: w345 -> [w349] mode=indexing
                n157 = local read "glitch (mil)"() -> (w346:dbl)
                n158 = Unbundle By Name(w349) -> ("D_giltch"=w348:ext)
                n159 = Greater?(x=w348, y=w346) -> (0:w347:bool)
                n160 = case shown="True" w347 {
                  frame False {
                  }
                  frame True {
                    n161 = local write "NG code"(1) -> ()
                  }
                }
              }
            }
          }
        }
        frame #2 {
          n162 = local read "NG code"() -> (w353:dbl)
          n163 = Equal To 0?(x=w353) -> (x = 0?=w352:bool)
          n164 = case shown="True" w352 {
            tunnel: w351 -> [_ w354]
            frame False {
            }
            frame True {
              n165 = for {
                tunnel: w354 -> [w357] mode=indexing
                n166 = local read "damaged (mil)"() -> (w355:dbl)
                n167 = Unbundle By Name(w357) -> ("D_damaged"=w358:ext)
                n168 = Greater?(x=w358, y=w355) -> (0:w356:bool)
                n169 = case shown="True" w356 {
                  frame False {
                  }
                  frame True {
                    n170 = local write "NG code"(3) -> ()
                  }
                }
              }
            }
          }
        }
        frame #3 {
          n171 = local read "NG code"() -> (w362:dbl)
          n172 = Equal To 0?(x=w362) -> (x = 0?=w361:bool)
          n173 = case shown="False" w361 {
            tunnel: w360 -> [_ w380]
            frame False {
            }
            frame True {
              n174 = Index Array(array=w380, index=2) -> (element=w376:ext)
              n175 = Index Array(array=w380, index=3) -> (element=w374:ext)
              n176 = Index Array(array=w380, index=0) -> (element=w377:ext)
              n177 = Index Array(array=w380, index=1) -> (element=w375:ext)
              n178 = Divide(x=w377, y=w376) -> (x/y=w371:ext)
              n179 = Divide(x=w375, y=w374) -> (x/y=w368:ext)
              n180 = Decrement(x=w368) -> (x-1=w369:ext)
              n181 = Decrement(x=w371) -> (x-1=w373:ext)
              n182 = Greater Than 0?(x=w369) -> (x > 0?=w370:bool)
              n183 = Greater Than 0?(x=w373) -> (x > 0?=w372:bool)
              n184 = local read "ratio (cutting offest)"() -> (w363:dbl)
              n185 = case shown="True" w370 {
                tunnel: w368 -> [w385 w387]
                tunnel: [w385 w386] -> w365
                frame False {
                }
                frame True {
                  n186 = Reciprocal(x=w387) -> (1/x=w386:ext)
                }
              }
              n187 = case shown="True" w372 {
                tunnel: w371 -> [w388 w390]
                tunnel: [w388 w389] -> w367
                frame False {
                }
                frame True {
                  n188 = Reciprocal(x=w390) -> (1/x=w389:ext)
                }
              }
              n189 = Less?(x=w367, y=w363) -> (x < y?=w366:bool)
              n190 = Less?(x=w365, y=w363) -> (x < y?=w364:bool)
              n191 = case shown="True" w366 {
                frame False {
                }
                frame True {
                  n192 = local write "NG code"(4) -> ()
                }
              }
              n193 = case shown="True" w364 {
                frame False {
                }
                frame True {
                  n194 = local write "NG code"(4) -> ()
                }
              }
            }
          }
        }
        frame #4 {
          n195 = local read "NG code"() -> (w392:dbl)
          n196 = Equal To 0?(x=w392) -> (x = 0?=w391:bool)
          n197 = case shown="True" w391 {
            frame False {
            }
            frame True {
            }
          }
        }
        frame #5 {
          n198 = local read "NG code"() -> (w394:dbl)
          n199 = Equal To 0?(x=w394) -> (x = 0?=w393:bool)
          n200 = local write "PASS"(w393) -> ()
          n201 = Tick Count (ms)() -> (millisecond timer value=w397:u32)
          n202 = Subtract(x=w397, y=w396) -> (x-y=→"time image processing":u32)
        }
      }
    }
  }
